vi "PM-A-Serial-read.vi"(5 "Max byte count per msg (50)":u32=50, 7 "sample rate [Hz] (1000)":dbl=1000.0, 8 "error in (no error)":errorcluster, 11 "VISA resource name in":refnum<visa-resource-name>) -> (0 "error out":errorcluster, 2 "data":waveform(dbl), 3 "VISA resource name out":refnum<visa-resource-name>)   [LabVIEW 2018]
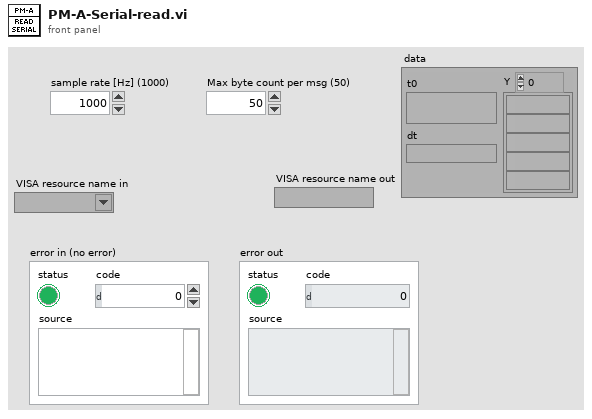
[diagram p1: front panel]
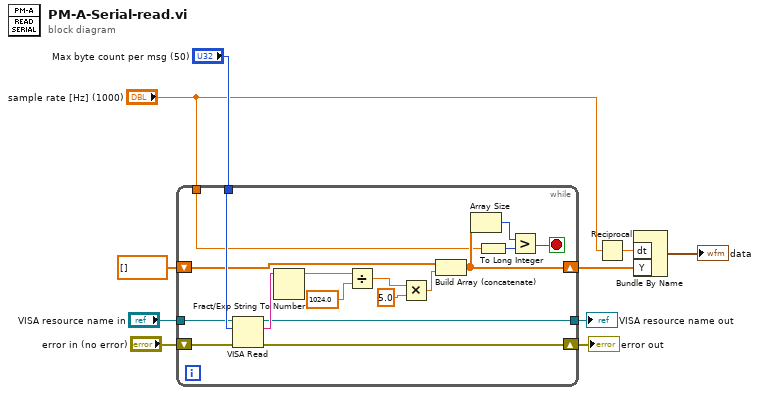
[diagram p0: block diagram]
diagram:
  n1 = while {
    tunnel: "Max byte count per msg (50)" -> [w27]
    shift-right: [w25] -> w8
    shift-left: "error in (no error)" -> [w26]
    shift-right: [w16] -> w4
    shift-left: dbl[] [] -> [w18]
    tunnel: "sample rate [Hz] (1000)" -> [w15]
    tunnel: "VISA resource name in" -> [w12]
    tunnel: [w11] -> w1
    stop <- w14 stop-if-true
    n2 = VISA Read(VISA resource name=w12, byte count=w27, error in (no error)=w26) -> (VISA resource name out=w11:refnum<visa-resource-name>, read buffer=w22:string, error out=w25:errorcluster)  [unwired: 1 out]
    n3 = Fract/Exp String To Number(string=w22) -> (number=w24:dbl)  [unwired: 3 in, 1 out]
    n4 = Divide(x=w24, y=1024.0) -> (x/y=w21:dbl)
    n5 = Multiply(x=w21, y=5.0) -> (x*y=w19:dbl)
    n6 = Build Array (concatenate)(w18, w19) -> (w16:dbl[])
    n7 = Array Size(array=w16) -> (size(s)=w17:i32)
    n8 = To Long Integer(number=w15) -> (32bit integer=w13:i32)
    n9 = Greater?(x=w17, y=w13) -> (0:w14:bool)
  }
  "error out" <- w8
  "VISA resource name out" <- w1
  n10 = Reciprocal(x="sample rate [Hz] (1000)") -> (1/x=w3:dbl)
  n11 = Bundle By Name("dt"=w3, "Y"=w4) -> (→"data":waveform(dbl))  [unwired: 1 in]
